vi "EnumToEnumAndLookup.vi"() -> ()   [LabVIEW 2024]
uses:
  SDL3/Render/PixelFormat--enum.ctl
  <vilib>/regexp/Match Regular Expression.xnode
  SDL3/Render/Render.lvlib
panel:
  out "Lookup":u32[](array[numeric]) format="%.0x"
  in  "#Define list":string="SDL_PIXELFORMAT_UNKNOWN = 0,\n    SDL_PIXELFORMAT_INDEX1LSB = 0x11100100u,\n        /* SDL_DEFINE_PIXELFORMAT(SDL_PIXELTYPE_INDEX1, SDL_BITMAPORDER_4321, 0, 1, 0), */\n    SDL_PIXELFORMAT_INDEX1MSB = 0x11200100u,\n        /* SDL_DEFINE_PIXELFORMAT(SDL_PIXELTYPE_INDEX1, SDL_BITMAPORDER_1234, 0, 1, 0), */\n    SDL_PIXELFORMAT_INDEX2LSB = 0x1c100200u,\n        /* SDL_DEFINE_PIXELFORMAT(SDL_PIXELTYPE_INDEX2, SDL_BITMAPORDER_4321, 0, 2, 0), */\n    SDL_PIXELFORMAT_INDEX2MSB = 0x1c200200u,\n        /* SDL_DEFINE_PIXELFORMAT(SDL_PIXELTYPE_INDEX2, SDL_BITMAPORDER_1234, 0, 2, 0), */\n    SDL_PIXELFORMAT_INDEX4LSB = 0x12100400u,\n        /* SDL_DEFINE_PIXELFORMAT(SDL_PIXELTYPE_INDEX4, SDL_BITMAPORDER_4321, 0, 4, 0), */\n    SDL_PIXELFORMAT_INDEX4MSB = 0x12200400u,\n        /* SDL_DEFINE_PIXELFORMAT(SDL_PIXELTYPE_INDEX4, SDL_BITMAPORDER_1234, 0, 4, 0), */\n    SDL_PIXELFORMAT_INDEX8 = 0x13000801u,\n        /* SDL_DEFINE_PIXELFORMAT(SDL_PIXELTYPE_INDEX8, 0, 0, 8, 1), */\n    SDL_PIXELFORMAT_RGB332 = 0x14110801u,\n        /* SDL_DEFINE_PIXELFORMAT(SDL_PIXELTYPE_PACKED8, SDL_PACKEDORDER_XRGB, SDL_PACKEDLAYOUT_332, 8, 1), */\n    SDL_PIXELFORMAT_XRGB4444 = 0x15120c02u,\n        /* SDL_DEFINE_PIXELFORMAT(SDL_PIXELTYPE_PACKED16, SDL_PACKEDORDER_XRGB, SDL_PACKEDLAYOUT_4444, 12, 2), */\n    SDL_PIXELFORMAT_XBGR4444 = 0x15520c02u,\n        /* SDL_DEFINE_PIXELFORMAT(SDL_PIXELTYPE_PACKED16, SDL_PACKEDORDER_XBGR, SDL_PACKEDLAYOUT_4444, 12, 2), */\n    SDL_PIXELFORMAT_XRGB1555 = 0x15130f02u,\n        /* SDL_DEFINE_PIXELFORMAT(SDL_PIXELTYPE_PACKED16, SDL_PACKEDORDER_XRGB, SDL_PACKEDLAYOUT_1555, 15, 2), */\n    SDL_PIXELFORMAT_XBGR1555 = 0x15530f02u,\n        /* SDL_DEFINE_PIXELFORMAT(SDL_PIXELTYPE_PACKED16, SDL_PACKEDORDER_XBGR, SDL_PACKEDLAYOUT_1555, 15, 2), */\n    SDL_PIXELFORMAT_ARGB4444 = 0x15321002u,\n        /* SDL_DEFINE_PIXELFORMAT(SDL_PIXELTYPE_PACKED16, SDL_PACKEDORDER_ARGB, SDL_PACKEDLAYOUT_4444, 16, 2), */\n    SDL_PIXELFORMAT_RGBA4444 = 0x15421002u,\n        /* SDL_DEFINE_PIXELFORMAT(SDL_PIXELTYPE_PACKED16, SDL_PACKEDORDER_RGBA, SDL_PACKEDLAYOUT_4444, 16, 2), */\n    SDL_PIXELFORMAT_ABGR4444 = 0x15721002u,\n        /* SDL_DEFINE_PIXELFORMAT(SDL_PIXELTYPE_PACKED16, SDL_PACKEDORDER_ABGR, SDL_PACKEDLAYOUT_4444, 16, 2), */\n    SDL_PIXELFORMAT_BGRA4444 = 0x15821002u,\n        /* SDL_DEFINE_PIXELFORMAT(SDL_PIXELTYPE_PACKED16, SDL_PACKEDORDER_BGRA, SDL_PACKEDLAYOUT_4444, 16, 2), */\n    SDL_PIXELFORMAT_ARGB1555 = 0x15331002u,\n        /* SDL_DEFINE_PIXELFORMAT(SDL_PIXELTYPE_PACKED16, SDL_PACKEDORDER_ARGB, SDL_PACKEDLAYOUT_1555, 16, 2), */\n    SDL_PIXELFORMAT_RGBA5551 = 0x15441002u,\n        /* SDL_DEFINE_PIXELFORMAT(SDL_PIXELTYPE_PACKED16, SDL_PACKEDORDER_RGBA, SDL_PACKEDLAYOUT_5551, 16, 2), */\n    SDL_PIXELFORMAT_ABGR1555 = 0x15731002u,\n        /* SDL_DEFINE_PIXELFORMAT(SDL_PIXELTYPE_PACKED16, SDL_PACKEDORDER_ABGR, SDL_PACKEDLAYOUT_1555, 16, 2), */\n    SDL_PIXELFORMAT_BGRA5551 = 0x15841002u,\n        /* SDL_DEFINE_PIXELFORMAT(SDL_PIXELTYPE_PACKED16, SDL_PACKEDORDER_BGRA, SDL_PACKEDLAYOUT_5551, 16, 2), */\n    SDL_PIXELFORMAT_RGB565 = 0x15151002u,\n        /* SDL_DEFINE_PIXELFORMAT(SDL_PIXELTYPE_PACKED16, SDL_PACKEDORDER_XRGB, SDL_PACKEDLAYOUT_565, 16, 2), */\n    SDL_PIXELFORMAT_BGR565 = 0x15551002u,\n        /* SDL_DEFINE_PIXELFORMAT(SDL_PIXELTYPE_PACKED16, SDL_PACKEDORDER_XBGR, SDL_PACKEDLAYOUT_565, 16, 2), */\n    SDL_PIXELFORMAT_RGB24 = 0x17101803u,\n        /* SDL_DEFINE_PIXELFORMAT(SDL_PIXELTYPE_ARRAYU8, SDL_ARRAYORDER_RGB, 0, 24, 3), */\n    SDL_PIXELFORMAT_BGR24 = 0x17401803u,\n        /* SDL_DEFINE_PIXELFORMAT(SDL_PIXELTYPE_ARRAYU8, SDL_ARRAYORDER_BGR, 0, 24, 3), */\n    SDL_PIXELFORMAT_XRGB8888 = 0x16161804u,\n        /* SDL_DEFINE_PIXELFORMAT(SDL_PIXELTYPE_PACKED32, SDL_PACKEDORDER_XRGB, SDL_PACKEDLAYOUT_8888, 24, 4), */\n    SDL_PIXELFORMAT_RGBX8888 = 0x16261804u,\n        /* SDL_DEFINE_PIXELFORMAT(SDL_PIXELTYPE_PACKED32, SDL_PACKEDORDER_RGBX, SDL_PACKEDLAYOUT_8888, 24, 4), */\n    SDL_PIXELFORMAT_XBGR8888 = 0x16561804u,\n        /* SDL_DEFINE_PIXELFORMAT(SDL_PIXELTYPE_PACKED32, SDL_PACKEDORDER_XBGR, SDL_PACKEDLAYOUT_8888, 24, 4), */\n    SDL_PIXELFORMAT_BGRX8888 = 0x16661804u,\n        /* SDL_DEFINE_PIXELFORMAT(SDL_PIXELTYPE_PACKED32, SDL_PACKEDORDER_BGRX, SDL_PACKEDLAYOUT_8888, 24, 4), */\n    SDL_PIXELFORMAT_ARGB8888 = 0x16362004u,\n        /* SDL_DEFINE_PIXELFORMAT(SDL_PIXELTYPE_PACKED32, SDL_PACKEDORDER_ARGB, SDL_PACKEDLAYOUT_8888, 32, 4), */\n    SDL_PIXELFORMAT_RGBA8888 = 0x16462004u,\n        /* SDL_DEFINE_PIXELFORMAT(SDL_PIXELTYPE_PACKED32, SDL_PACKEDORDER_RGBA, SDL_PACKEDLAYOUT_8888, 32, 4), */\n    SDL_PIXELFORMAT_ABGR8888 = 0x16762004u,\n        /* SDL_DEFINE_PIXELFORMAT(SDL_PIXELTYPE_PACKED32, SDL_PACKEDORDER_ABGR, SDL_PACKEDLAYOUT_8888, 32, 4), */\n    SDL_PIXELFORMAT_BGRA8888 = 0x16862004u,\n        /* SDL_DEFINE_PIXELFORMAT(SDL_PIXELTYPE_PACKED32, SDL_PACKEDORDER_BGRA, SDL_PACKEDLAYOUT_8888, 32, 4), */\n    SDL_PIXELFORMAT_XRGB2101010 = 0x16172004u,\n        /* SDL_DEFINE_PIXELFORMAT(SDL_PIXELTYPE_PACKED32, SDL_PACKEDORDER_XRGB, SDL_PACKEDLAYOUT_2101010, 32, 4), */\n    SDL_PIXELFORMAT_XBGR2101010 = 0x16572004u,\n        /* SDL_DEFINE_PIXELFORMAT(SDL_PIXELTYPE_PACKED32, SDL_PACKEDORDER_XBGR, SDL_PACKEDLAYOUT_2101010, 32, 4), */\n    SDL_PIXELFORMAT_ARGB2101010 = 0x16372004u,\n        /* SDL_DEFINE_PIXELFORMAT(SDL_PIXELTYPE_PACKED32, SDL_PACKEDORDER_ARGB, SDL_PACKEDLAYOUT_2101010, 32, 4), */\n    SDL_PIXELFORMAT_ABGR2101010 = 0x16772004u,\n        /* SDL_DEFINE_PIXELFORMAT(SDL_PIXELTYPE_PACKED32, SDL_PACKEDORDER_ABGR, SDL_PACKEDLAYOUT_2101010, 32, 4), */\n    SDL_PIXELFORMAT_RGB48 = 0x18103006u,\n        /* SDL_DEFINE_PIXELFORMAT(SDL_PIXELTYPE_ARRAYU16, SDL_ARRAYORDER_RGB, 0, 48, 6), */\n    SDL_PIXELFORMAT_BGR48 = 0x18403006u,\n        /* SDL_DEFINE_PIXELFORMAT(SDL_PIXELTYPE_ARRAYU16, SDL_ARRAYORDER_BGR, 0, 48, 6), */\n    SDL_PIXELFORMAT_RGBA64 = 0x18204008u,\n        /* SDL_DEFINE_PIXELFORMAT(SDL_PIXELTYPE_ARRAYU16, SDL_ARRAYORDER_RGBA, 0, 64, 8), */\n    SDL_PIXELFORMAT_ARGB64 = 0x18304008u,\n        /* SDL_DEFINE_PIXELFORMAT(SDL_PIXELTYPE_ARRAYU16, SDL_ARRAYORDER_ARGB, 0, 64, 8), */\n    SDL_PIXELFORMAT_BGRA64 = 0x18504008u,\n        /* SDL_DEFINE_PIXELFORMAT(SDL_PIXELTYPE_ARRAYU16, SDL_ARRAYORDER_BGRA, 0, 64, 8), */\n    SDL_PIXELFORMAT_ABGR64 = 0x18604008u,\n        /* SDL_DEFINE_PIXELFORMAT(SDL_PIXELTYPE_ARRAYU16, SDL_ARRAYORDER_ABGR, 0, 64, 8), */\n    SDL_PIXELFORMAT_RGB48_FLOAT = 0x1a103006u,\n        /* SDL_DEFINE_PIXELFORMAT(SDL_PIXELTYPE_ARRAYF16, SDL_ARRAYORDER_RGB, 0, 48, 6), */\n    SDL_PIXELFORMAT_BGR48_FLOAT = 0x1a403006u,\n        /* SDL_DEFINE_PIXELFORMAT(SDL_PIXELTYPE_ARRAYF16, SDL_ARRAYORDER_BGR, 0, 48, 6), */\n    SDL_PIXELFORMAT_RGBA64_FLOAT = 0x1a204008u,\n        /* SDL_DEFINE_PIXELFORMAT(SDL_PIXELTYPE_ARRAYF16, SDL_ARRAYORDER_RGBA, 0, 64, 8), */\n    SDL_PIXELFORMAT_ARGB64_FLOAT = 0x1a304008u,\n        /* SDL_DEFINE_PIXELFORMAT(SDL_PIXELTYPE_ARRAYF16, SDL_ARRAYORDER_ARGB, 0, 64, 8), */\n    SDL_PIXELFORMAT_BGRA64_FLOAT = 0x1a504008u,\n        /* SDL_DEFINE_PIXELFORMAT(SDL_PIXELTYPE_ARRAYF16, SDL_ARRAYORDER_BGRA, 0, 64, 8), */\n    SDL_PIXELFORMAT_ABGR64_FLOAT = 0x1a604008u,\n        /* SDL_DEFINE_PIXELFORMAT(SDL_PIXELTYPE_ARRAYF16, SDL_ARRAYORDER_ABGR, 0, 64, 8), */\n    SDL_PIXELFORMAT_RGB96_FLOAT = 0x1b10600cu,\n        /* SDL_DEFINE_PIXELFORMAT(SDL_PIXELTYPE_ARRAYF32, SDL_ARRAYORDER_RGB, 0, 96, 12), */\n    SDL_PIXELFORMAT_BGR96_FLOAT = 0x1b40600cu,\n        /* SDL_DEFINE_PIXELFORMAT(SDL_PIXELTYPE_ARRAYF32, SDL_ARRAYORDER_BGR, 0, 96, 12), */\n    SDL_PIXELFORMAT_RGBA128_FLOAT = 0x1b208010u,\n        /* SDL_DEFINE_PIXELFORMAT(SDL_PIXELTYPE_ARRAYF32, SDL_ARRAYORDER_RGBA, 0, 128, 16), */\n    SDL_PIXELFORMAT_ARGB128_FLOAT = 0x1b308010u,\n        /* SDL_DEFINE_PIXELFORMAT(SDL_PIXELTYPE_ARRAYF32, SDL_ARRAYORDER_ARGB, 0, 128, 16), */\n    SDL_PIXELFORMAT_BGRA128_FLOAT = 0x1b508010u,\n        /* SDL_DEFINE_PIXELFORMAT(SDL_PIXELTYPE_ARRAYF32, SDL_ARRAYORDER_BGRA, 0, 128, 16), */\n    SDL_PIXELFORMAT_ABGR128_FLOAT = 0x1b608010u,\n        /* SDL_DEFINE_PIXELFORMAT(SDL_PIXELTYPE_ARRAYF32, SDL_ARRAYORDER_ABGR, 0, 128, 16), */\n\n    SDL_PIXELFORMAT_YV12 = 0x32315659u,      /**< Planar mode: Y + V + U  (3 planes) */\n        /* SDL_DEFINE_PIXELFOURCC('Y', 'V', '1', '2'), */\n    SDL_PIXELFORMAT_IYUV = 0x56555949u,      /**< Planar mode: Y + U + V  (3 planes) */\n        /* SDL_DEFINE_PIXELFOURCC('I', 'Y', 'U', 'V'), */\n    SDL_PIXELFORMAT_YUY2 = 0x32595559u,      /**< Packed mode: Y0+U0+Y1+V0 (1 plane) */\n        /* SDL_DEFINE_PIXELFOURCC('Y', 'U', 'Y', '2'), */\n    SDL_PIXELFORMAT_UYVY = 0x59565955u,      /**< Packed mode: U0+Y0+V0+Y1 (1 plane) */\n        /* SDL_DEFINE_PIXELFOURCC('U', 'Y', 'V', 'Y'), */\n    SDL_PIXELFORMAT_YVYU = 0x55595659u,      /**< Packed mode: Y0+V0+Y1+U0 (1 plane) */\n        /* SDL_DEFINE_PIXELFOURCC('Y', 'V', 'Y', 'U'), */\n    SDL_PIXELFORMAT_NV12 = 0x3231564eu,      /**< Planar mode: Y + U/V interleaved  (2 planes) */\n        /* SDL_DEFINE_PIXELFOURCC('N', 'V', '1', '2'), */\n    SDL_PIXELFORMAT_NV21 = 0x3132564eu,      /**< Planar mode: Y + V/U interleaved  (2 planes) */\n        /* SDL_DEFINE_PIXELFOURCC('N', 'V', '2', '1'), */\n    SDL_PIXELFORMAT_P010 = 0x30313050u,      /**< Planar mode: Y + U/V interleaved  (2 planes) */\n        /* SDL_DEFINE_PIXELFOURCC('P', '0', '1', '0'), */\n    SDL_PIXELFORMAT_EXTERNAL_OES = 0x2053454fu,     /**< Android video texture format */\n        /* SDL_DEFINE_PIXELFOURCC('O', 'E', 'S', ' ') */"
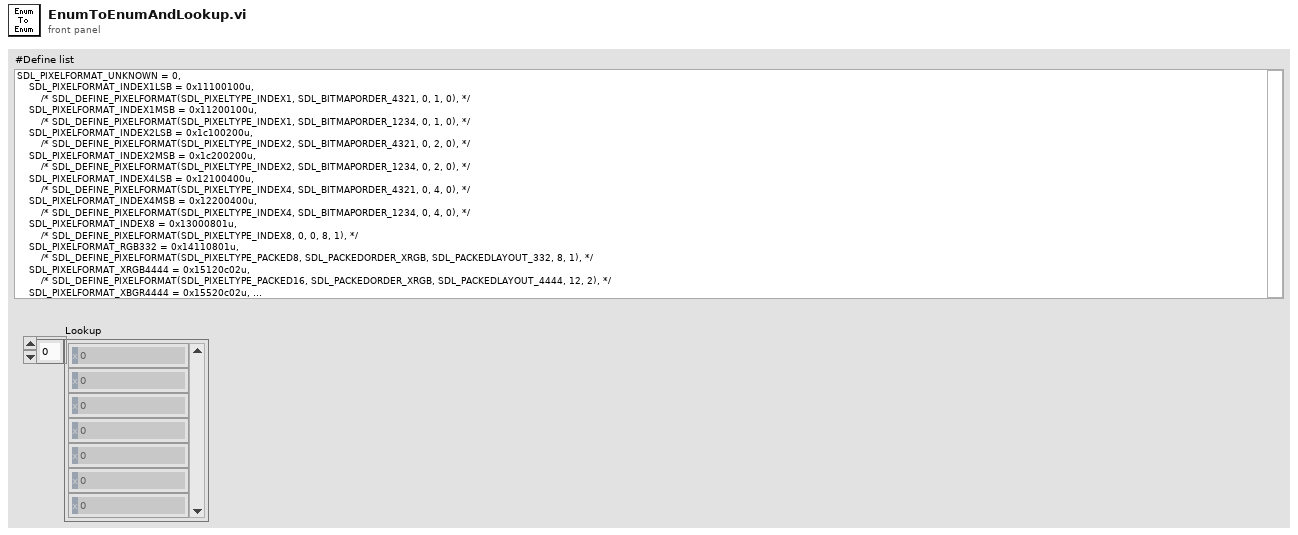
[diagram p1: front panel]
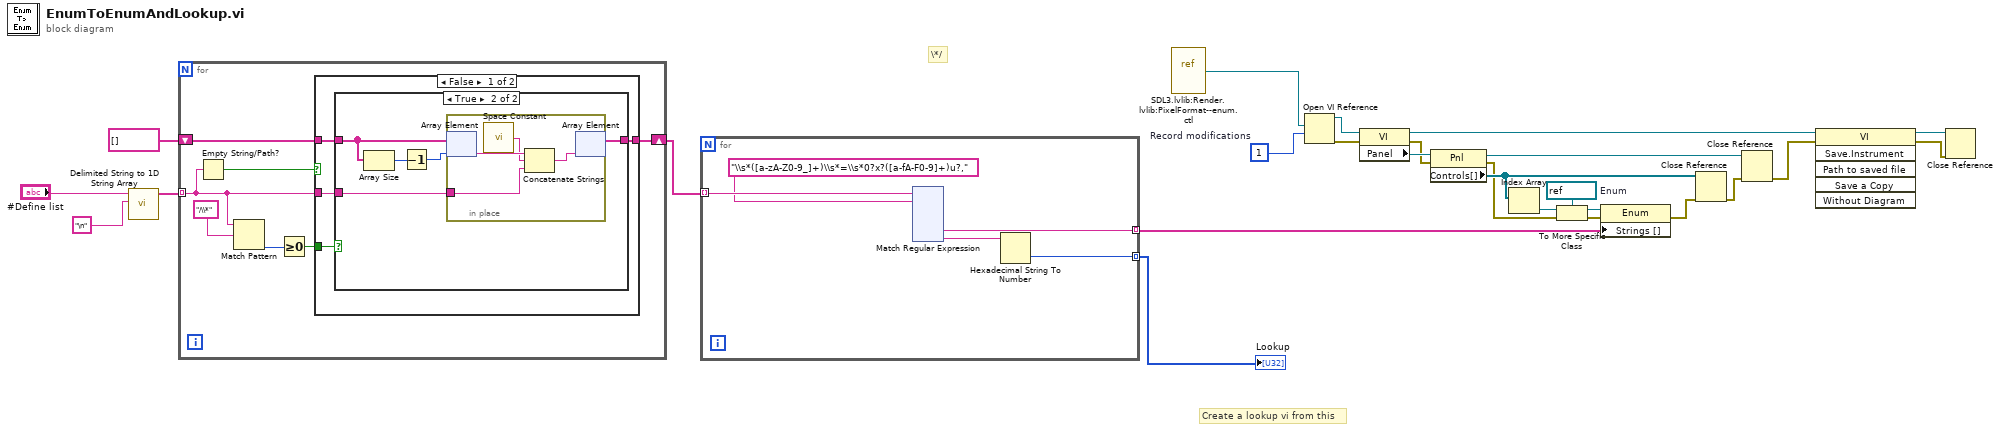
[diagram p0: block diagram]
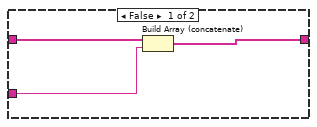
[diagram p2: hidden frame]
diagram:
  w13 = refnum<vi> refnum  # Enum
  w19 = 1  # Record modifications
  # "Create a lookup vi from this"
  # "\\*/"
  n1 = call <vilib>:"Delimited String to 1D String Array.vi"("delimiter"="\n", "delimited string"="#Define list") -> ("string array"=w24:string[])  [unwired: 9 in]
  n2 = for {
    tunnel: w24 -> [w28] mode=indexing
    shift-right: [w31] -> w22
    shift-left: string[] [] -> [w32]
    n3 = Empty String/Path?(string/path=w28) -> (empty?=w27:bool)
    n4 = Match Pattern(string=w28, regular expression="/\\*") -> (offset past match=w30:i32)  [unwired: 1 in, 3 out]
    n5 = Greater Or Equal To 0?(x=w30) -> (x >= 0?=w29:bool)
    n6 = case shown="False" w27 {
      tunnel: w32 -> [w37 w50]
      tunnel: [w36 w50] -> w31
      tunnel: w29 -> [w35 _]
      tunnel: w28 -> [w34 _]
      frame False {
        n7 = case shown="True" w35 {
          tunnel: w37 -> [w40 w45]
          tunnel: [w39 w44] -> w36
          tunnel: w34 -> [w38 w43]
          frame False {
            n8 = Build Array (concatenate)(w40, w38) -> (w39:string[])
          }
          frame True {
            n9 = Array Size(array=w45) -> (size(s)=w42:i32)
            n10 = Decrement(x=w42) -> (x-1=w41:i32)
            n11 = in-place {
              in-place-border: w43 -> [w46]
              n12 = in-place-array #1(w45, w41) -> (w49:string)
              n13 = call <vilib>:"Space Constant.vi"() -> ("String"=w47:string)
              n14 = Concatenate Strings(w49, w47, w46) -> (w48:string)
              n15 = in-place-array #1(w48) -> (w44:string[])  [unwired: 1 out]
            }
          }
        }
      }
      frame True {
      }
    }
  }
  n16 = for {
    tunnel: w22 -> [w55] mode=indexing
    tunnel: [w52] -> w1 mode=indexing
    tunnel: [w51] -> w3 mode=indexing
    n17 = xnode "Match Regular Expression"("input string"=w55, "regular expression"="\\s*([a-zA-Z0-9_]+)\\s*=\\s*0?x?([a-fA-F0-9]+)u?,") -> ("submatch 1"=w51:string, "submatch 2"=w53:string)  [unwired: 4 in, 5 out]
    n18 = Hexadecimal String To Number(string=w53) -> (number=w52:u32)  [unwired: 2 in, 1 out]
  }
  "Lookup" <- w1
  n19 = vi-ref "SDL3.lvlib:Render.lvlib:PixelFormat--enum.ctl"() -> (w20:refnum<vi>)
  n20 = Open VI Reference(vi path=w20, options=w19) -> (vi reference=w18:refnum<vi>, error out=w21:errorcluster)  [unwired: 4 in]
  n21 = property class="VI"(reference=w18, error in=w21) -> (reference out=w8:refnum<vi>, error out=w16:errorcluster, "Panel"=w17:refnum<vi>)
  n22 = property class="Pnl"(reference=w17, error in=w16) -> (reference out=w15:refnum<vi>, error out=w6:errorcluster, "Controls[]"=w11:refnum<vi>[])
  n23 = Index Array(array=w11) -> (element=w12:refnum<vi>)  [unwired: 1 in]
  n24 = To More Specific Class(target class=w13, reference=w12, error in=w6) -> (specific class reference=w5:refnum<vi>, error out=w4:errorcluster)
  n25 = property class="Enum"(reference=w5, error in=w4, "Strings []"=w3) -> (error out=w2:errorcluster)  [unwired: 1 out]
  n26 = Close Reference(reference=w11, error in (no error)=w2) -> (error out=w10:errorcluster)
  n27 = Close Reference(reference=w15, error in (no error)=w10) -> (error out=w14:errorcluster)
  n28 = invoke class="VI" method="Save.Instrument"(reference=w8, error in=w14) -> (reference out=w7:refnum<vi>, error out=w9:errorcluster)  [unwired: 4 in, 4 out]
  n29 = Close Reference(reference=w7, error in (no error)=w9) -> ()  [unwired: 1 out]
